vi "rename channel.vi"(8 "error in":errorcluster, 9 "new name":string, 10 "old name":string, 11 "sample module configuration in":refnum<class "sample module configuration.lvclass">) -> (0 "error out":errorcluster, 3 "sample module configuration out":refnum<class "sample module configuration.lvclass">)   [LabVIEW 2013, in "sample module configuration.lvclass"]
uses:
  sample module configuration.lvclass
  sample module configuration.lvclass/sample module configuration.ctl
  <vilib>/NI/Tag Bus/tag/tag descriptor.lvclass/tag descriptor.ctl
  <vilib>/NI/Tag Bus/tag/read tag name.vi
  <vilib>/NI/Tag Bus/tag/tag descriptor.lvclass
  root configuration/TBM configuration.lvclass
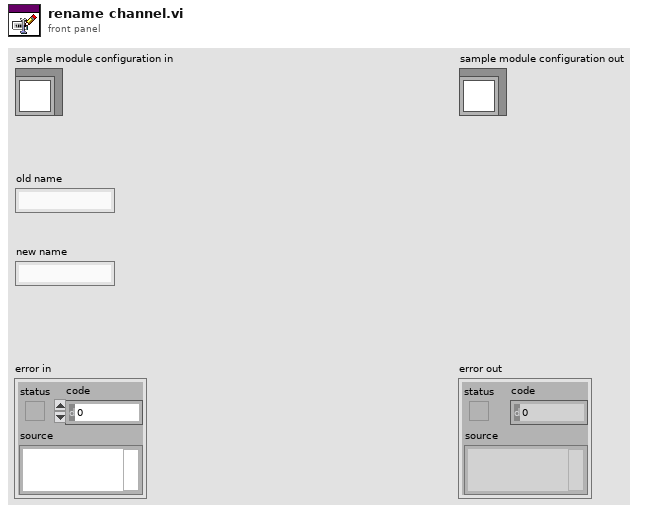
[diagram p1: front panel]
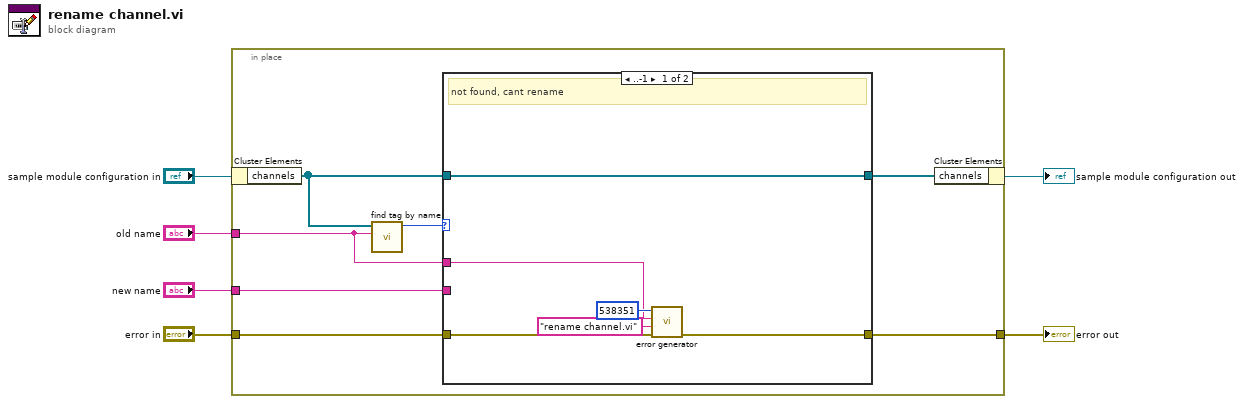
[diagram p0: block diagram]
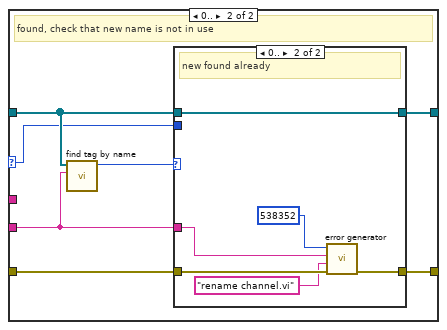
[diagram p2: hidden frame]
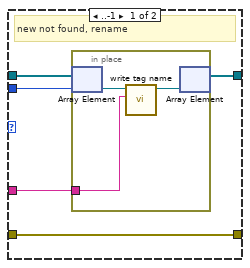
[diagram p3: hidden frame]
diagram:
  n1 = in-place {
    in-place-border: "old name" -> [w11]
    in-place-border: "new name" -> [w7]
    in-place-border: [w10] -> w2
    in-place-border: "error in" -> [w8]
    n2 = in-place-cluster #1("sample module configuration in") -> ("channels"=w12:refnum<class "TBM channel.lvclass">[])
    n3 = call <vilib>:"find tag by name.vi"("name"=w11, "tags in"=w12) -> ("index"=w13:i32)  [unwired: 9 in]
    n4 = case shown="..-1" w13 {
      selector: w13 -> [_ w20]
      tunnel: w12 -> [w16 w25]
      tunnel: w11 -> [w18 _]
      tunnel: [w17 w21] -> w10
      tunnel: [w16 w26] -> w9
      tunnel: w8 -> [w15 w22]
      tunnel: w7 -> [_ w24]
      frame ..-1 {
        # "not found, cant rename"
        n5 = call "error generator.vi"("error in"=w15, "source"="rename channel.vi", "append error message"=w18, "error code (0)"=538351) -> ("error out"=w17:errorcluster)  [unwired: 7 in]
      }
      frame 0.. {
        # "found, check that new name is not in use"
        n6 = call <vilib>:"find tag by name.vi"("name"=w24, "tags in"=w25) -> ("index"=w23:i32)  [unwired: 9 in]
        n7 = case shown="0.." w23 {
          tunnel: [w31 w40] -> w26
          tunnel: w20 -> [w30 _]
          tunnel: w25 -> [w29 w40]
          tunnel: w24 -> [w28 w36]
          tunnel: w22 -> [w27 w38]
          tunnel: [w27 w39] -> w21
          frame ..-1 {
            # "new not found, rename"
            n8 = in-place {
              in-place-border: w28 -> [w32]
              n9 = in-place-array #2(w29, w30) -> (w34:refnum<class "TBM channel.lvclass">)
              n10 = call <vilib>:"write tag name.vi"("name"=w32, "system tag in"=w34) -> ("system tag out"=w33:refnum<class "TBM channel.lvclass">)  [unwired: 8 in, 1 out]
              n11 = in-place-array #2(w33) -> (w31:refnum<class "TBM channel.lvclass">[])  [unwired: 1 out]
            }
          }
          frame 0.. {
            # "new found already"
            n12 = call "error generator.vi"("error in"=w38, "source"="rename channel.vi", "append error message"=w36, "error code (0)"=538352) -> ("error out"=w39:errorcluster)  [unwired: 7 in]
          }
        }
      }
    }
    n13 = in-place-cluster #1("channels"=w9) -> (→"sample module configuration out":refnum<class "sample module configuration.lvclass">)
  }
  "error out" <- w2
